vi "PImitStör.vi"(10 "a":dbl) -> (2 "F":dbl)   [LabVIEW 2013]
uses:
  <vilib>/Simulation/Implementation/Shared/SIMSCR Execution Mode.ctl
  <vilib>/Simulation/Scripting/Companion Diagram/SimConfigNode/SimParams.ctl
  <vilib>/Simulation/Scripting/Companion Diagram/SimConfigNode/_simSolvers.ctl
  <vilib>/Simulation/Param Hierarchy/Typedefs/SIMPH Param Control Actions.ctl
  <vilib>/Simulation/Implementation/Shared/SIM limit type.ctl
  <vilib>/Simulation/Implementation/Shared/NILVSim_ParamChanged.vi
  <vilib>/Simulation/Implementation/Shared/NILVSIM_BeginStep.vi
  <vilib>/Simulation/SignalArithmetic/Implementation/NILVSim Gain.llb/SIM Gain (scalar).vi
  <vilib>/Simulation/ContinuousLinear/Implementation/NILVSim Integrator new.llb/SIM Integrator distributor (scalar).vi
  <vilib>/Simulation/ContinuousLinear/Implementation/NILVSim Derivative.llb/SIM derivative (scalar).vi
  <vilib>/Simulation/Nonlinear/Implementation/NILVSim Saturation.llb/SIM Saturation (scalar).vi
  <vilib>/Simulation/ContinuousLinear/Implementation/NILVSim ZeroPoleGain Direct.llb/SIM  ZeroPoleGain Direct (SISO).vi
  <vilib>/Simulation/ContinuousLinear/Implementation/NILVSim Integrator new.llb/SIM Integrator collector (scalar).vi
  <vilib>/Simulation/Implementation/Shared/NILVSim_Manager.vi
  <vilib>/Simulation/Implementation/Shared/NILVSim_FinalizeModel.vi
  <vilib>/Simulation/Implementation/Shared/SIM Unbundle Sim Info.vi
  <vilib>/Utility/error.llb/Clear Errors.vi
  <vilib>/Simulation/Implementation/Shared/NILVSim_GetModelError.vi
  <vilib>/Simulation/Implementation/Shared/SIM SimErrorHandler.vi
  <vilib>/Simulation/Implementation/Shared/SIM Bundle Sim Info.vi
  <vilib>/Simulation/Implementation/Shared/SIMSH Read Queue.vi
  <vilib>/Simulation/Implementation/Shared/NILVSim_Initialize.vi
  <vilib>/Simulation/Utility/Implementation/NILVSim Get Time and IsAcceptedStep.vi
  <vilib>/Simulation/Scripting/Companion Diagram/SimConfigNode/SimDog.xnode
  <vilib>/Simulation/Implementation/XNodeFramework/SimXNode/SimX.xnode
  <vilib>/Simulation/ContinuousLinear/Implementation/NILVSim Integrator new.llb/SIM Integrator (scalar).vi
  <vilib>/Simulation/Implementation/Shared/NI_SIM_Implementation.lvlib
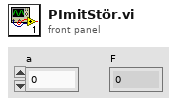
[diagram p1: front panel]
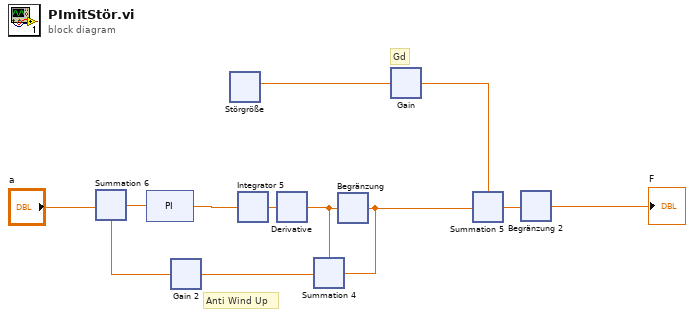
[diagram p0: block diagram]
diagram:
  # "Anti Wind Up"
  # "Gd"
  n1 = xnode "Störgröße"() -> ("Fsx"=w10:dbl)  [unwired: 11 out]
  n2 = xnode ("Gain")("input"=w10) -> ("output"=w4:dbl)  [unwired: 3 in]
  n3 = xnode ("Summation 6")("Operand1"="a", "Operand2"=w3) -> ("Result"=w2:dbl)
  n4 = xnode "PI"("input u(t)"=w2) -> ("output y(t)"=w5:dbl)  [unwired: 4 in, 1 out]
  n5 = xnode ("Integrator 5")("input"=w5) -> ("output"=w1:dbl)  [unwired: 9 in, 2 out]
  n6 = xnode ("Derivative")("input"=w1) -> ("output"=w6:dbl)  [unwired: 2 in]
  n7 = xnode ("Begränzung")("input"=w6) -> ("output"=w9:dbl)  [unwired: 4 in]
  n8 = xnode ("Summation 4")("Operand1"=w6, "Operand2"=w9) -> ("Result"=w7:dbl)
  n9 = xnode ("Gain 2")("input"=w7) -> ("output"=w3:dbl)  [unwired: 3 in]
  n10 = xnode ("Summation 5")("Operand1"=w4, "Operand2"=w9) -> ("Result"=w8:dbl)
  n11 = xnode ("Begränzung 2")("input"=w8) -> ("output"=→"F":dbl)  [unwired: 4 in]
